vi "Benchmark SV Send  LV2012 - NI Verified - 1000 Byte - 1Var.vi"() -> ()   [LabVIEW 2019]
uses:
  <vilib>/Platform/TimedLoop/XDataNode/timing_clust.ctl
  <vilib>/Platform/TimedLoop/XDataNode/nitl_modes.ctl
  <vilib>/Platform/TimedLoop/XDataNode/wakeup.ctl
  <vilib>/platform/TimedLoop/XDataNode/XDataNode.xnode
  <vilib>/Platform/TimedLoop/XDataNode/XDNodeRunTimeDep.lvlib
panel:
  in  "Client Closed":string="The client VI closed the connection."
  in  "Stop":bool
  out "Time":u32
  out "Tries":u32
  out "Average Delay (ms)":dbl
  out "Delay (ms)":u32
  # "Overview:  Coding that exemplifies how to benchmark the communication of Shared Variables.\nRequirements: LabVIEW 2012 or compatible\nInstructions:\n1.  Run the \"Benchmark SV Receive LV2012 - NI Verified.vi\"\n2. Run this VI\n3. Watch the amount of time it takes to communicate\n4. Stop both VIs"
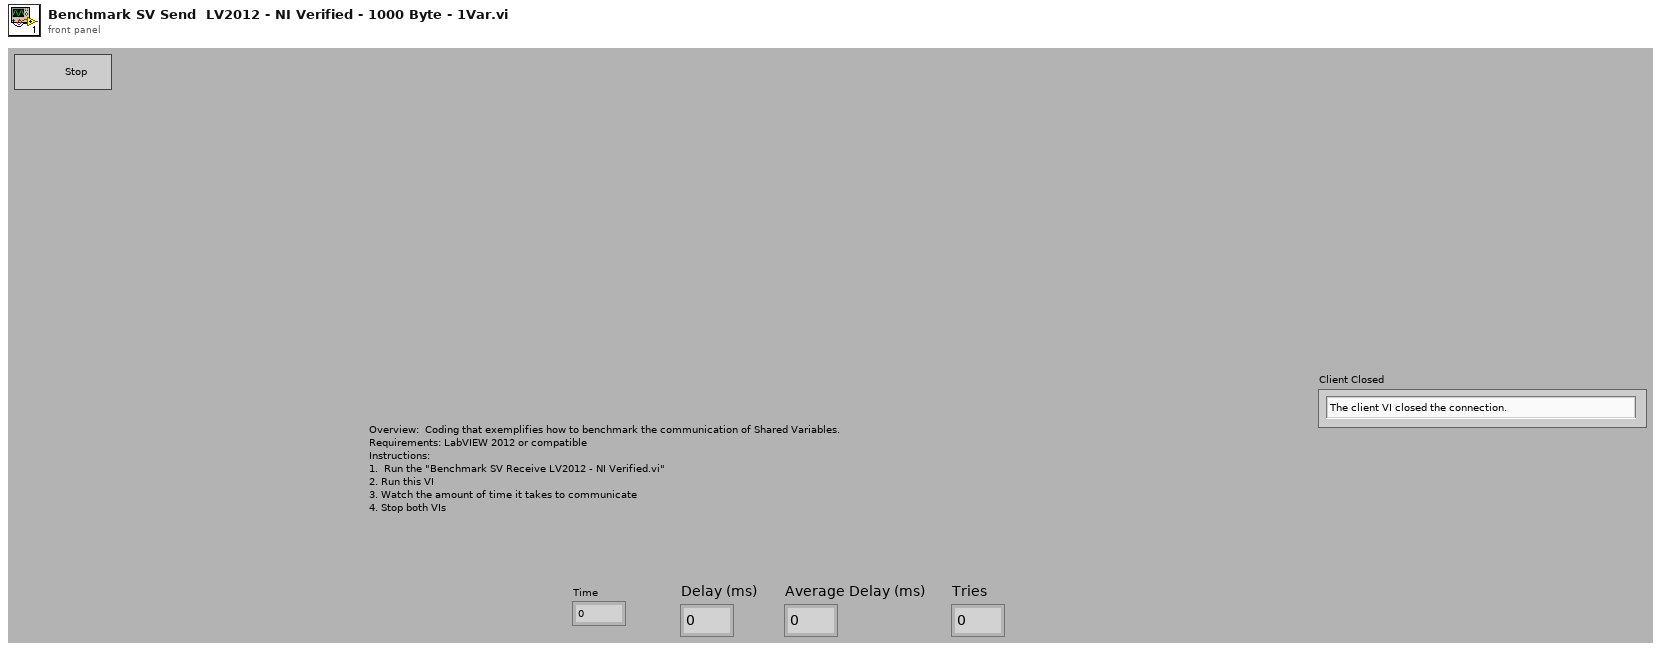
[diagram p1: front panel]
types:
  T1 = typedef "XDNodeRunTimeDep.lvlib/timing_clust.ctl" = cluster{"Expected End [f-1]":u64, "Actual End [f-1]":u64, "Finished Late? [f-1]":bool, "Expected End [i-1]":u64, "Actual End [i-1]":u64, "Finished Late? [i-1]":bool, "Expected Start [i]":u64, "Actual Start [i]":u64, "Expected Start [f]":u64, "Actual Start [f]":u64, "Source Name":string, "Structure Name":string, "Period":i64, "Deadline":i64, "Offset":i64, "Start":i64, "Priority":i32, "Timeout":i32, "Mode":T2, "Wakeup Reason":T3, "Error":errorcluster, "Source Type":string, "Secondary Source Type":string, "Global End Time":u64, "Global Start Time":u64, "Frame Duration":u64, "Iteration Duration":u64, "Assigned CPU":i32, "I/O Scan Engine Mode":u32}
  T2 = typedef "XDNodeRunTimeDep.lvlib/nitl_modes.ctl" = enum32{"No Change", "Process missed periods, maintain original phase", "Discard missed periods, maintain original phase", "Process missed periods, ignore original phase", "Discard missed periods, ignore original phase"}
  T3 = typedef "XDNodeRunTimeDep.lvlib/wakeup.ctl" = enum32{"Normal", "Aborted", "Asynchronous wakeup", "Timing source error", "Timed loop error", "Timeout"}
  T4 = cluster{i32, i32, i32, i32, i32, i32, i32, i32, i32, i32, i32, i32, i32, i32, i32, i32, i32, i32, i32, i32}
  T5 = cluster{cluster{i32, i32, i32, i32, i32, i32, i32, i32, i32, i32, i32, i32, i32, i32, i32, i32, i32, i32, i32, i32}, cluster{i32, i32, i32, i32, i32, i32, i32, i32, i32, i32, i32, i32, i32, i32, i32, i32, i32, i32, i32, i32}, cluster{i32, i32, i32, i32, i32, i32, i32, i32, i32, i32, i32, i32, i32, i32, i32, i32, i32, i32, i32, i32}, cluster{i32, i32, i32, i32, i32, i32, i32, i32, i32, i32, i32, i32, i32, i32, i32, i32, i32, i32, i32, i32}, cluster{i32, i32, i32, i32, i32, i32, i32, i32, i32, i32, i32, i32, i32, i32, i32, i32, i32, i32, i32, i32}, cluster{i32, i32, i32, i32, i32, i32, i32, i32, i32, i32, i32, i32, i32, i32, i32, i32, i32, i32, i32, i32}, cluster{i32, i32, i32, i32, i32, i32, i32, i32, i32, i32, i32, i32, i32, i32, i32, i32, i32, i32, i32, i32}, cluster{i32, i32, i32, i32, i32, i32, i32, i32, i32, i32, i32, i32, i32, i32, i32, i32, i32, i32, i32, i32}, cluster{i32, i32, i32, i32, i32, i32, i32, i32, i32, i32, i32, i32, i32, i32, i32, i32, i32, i32, i32, i32}, cluster{i32, i32, i32, i32, i32, i32, i32, i32, i32, i32, i32, i32, i32, i32, i32, i32, i32, i32, i32, i32}, cluster{i32, i32, i32, i32, i32, i32, i32, i32, i32, i32, i32, i32, i32, i32, i32, i32, i32, i32, i32, i32}, cluster{i32, i32, i32, i32, i32, i32, i32, i32, i32, i32, i32, i32, i32, i32, i32, i32, i32, i32, i32, i32}, cluster{i32, i32, i32, i32, i32, i32, i32, i32, i32, i32, i32, i32, i32, i32, i32, i32, i32, i32, i32, i32}, cluster{i32, i32, i32, i32, i32, i32, i32, i32, i32, i32, i32, i32, i32, i32, i32, i32, i32, i32, i32, i32}, cluster{i32, i32, i32, i32, i32, i32, i32, i32, i32, i32, i32, i32, i32, i32, i32, i32, i32, i32, i32, i32}, cluster{i32, i32, i32, i32, i32, i32, i32, i32, i32, i32, i32, i32, i32, i32, i32, i32, i32, i32, i32, i32}, cluster{i32, i32, i32, i32, i32, i32, i32, i32, i32, i32, i32, i32, i32, i32, i32, i32, i32, i32, i32, i32}, cluster{i32, i32, i32, i32, i32, i32, i32, i32, i32, i32, i32, i32, i32, i32, i32, i32, i32, i32, i32, i32}, cluster{i32, i32, i32, i32, i32, i32, i32, i32, i32, i32, i32, i32, i32, i32, i32, i32, i32, i32, i32, i32}, cluster{i32, i32, i32, i32, i32, i32, i32, i32, i32, i32, i32, i32, i32, i32, i32, i32, i32, i32, i32, i32}, cluster{i32, i32, i32, i32, i32, i32, i32, i32, i32, i32, i32, i32, i32, i32, i32, i32, i32, i32, i32, i32}, cluster{i32, i32, i32, i32, i32, i32, i32, i32, i32, i32, i32, i32, i32, i32, i32, i32, i32, i32, i32, i32}, cluster{i32, i32, i32, i32, i32, i32, i32, i32, i32, i32, i32, i32, i32, i32, i32, i32, i32, i32, i32, i32}, cluster{i32, i32, i32, i32, i32, i32, i32, i32, i32, i32, i32, i32, i32, i32, i32, i32, i32, i32, i32, i32}, cluster{i32, i32, i32, i32, i32, i32, i32, i32, i32, i32, i32, i32, i32, i32, i32, i32, i32, i32, i32, i32}, cluster{i32, i32, i32, i32, i32, i32, i32, i32, i32, i32, i32, i32, i32, i32, i32, i32, i32, i32, i32, i32}, cluster{i32, i32, i32, i32, i32, i32, i32, i32, i32, i32, i32, i32, i32, i32, i32, i32, i32, i32, i32, i32}, cluster{i32, i32, i32, i32, i32, i32, i32, i32, i32, i32, i32, i32, i32, i32, i32, i32, i32, i32, i32, i32}, cluster{i32, i32, i32, i32, i32, i32, i32, i32, i32, i32, i32, i32, i32, i32, i32, i32, i32, i32, i32, i32}, cluster{i32, i32, i32, i32, i32, i32, i32, i32, i32, i32, i32, i32, i32, i32, i32, i32, i32, i32, i32, i32}, cluster{i32, i32, i32, i32, i32, i32, i32, i32, i32, i32, i32, i32, i32, i32, i32, i32, i32, i32, i32, i32}, cluster{i32, i32, i32, i32, i32, i32, i32, i32, i32, i32, i32, i32, i32, i32, i32, i32, i32, i32, i32, i32}, cluster{i32, i32, i32, i32, i32, i32, i32, i32, i32, i32, i32, i32, i32, i32, i32, i32, i32, i32, i32, i32}, cluster{i32, i32, i32, i32, i32, i32, i32, i32, i32, i32, i32, i32, i32, i32, i32, i32, i32, i32, i32, i32}, cluster{i32, i32, i32, i32, i32, i32, i32, i32, i32, i32, i32, i32, i32, i32, i32, i32, i32, i32, i32, i32}, cluster{i32, i32, i32, i32, i32, i32, i32, i32, i32, i32, i32, i32, i32, i32, i32, i32, i32, i32, i32, i32}, cluster{i32, i32, i32, i32, i32, i32, i32, i32, i32, i32, i32, i32, i32, i32, i32, i32, i32, i32, i32, i32}, cluster{i32, i32, i32, i32, i32, i32, i32, i32, i32, i32, i32, i32, i32, i32, i32, i32, i32, i32, i32, i32}, cluster{i32, i32, i32, i32, i32, i32, i32, i32, i32, i32, i32, i32, i32, i32, i32, i32, i32, i32, i32, i32}, cluster{i32, i32, i32, i32, i32, i32, i32, i32, i32, i32, i32, i32, i32, i32, i32, i32, i32, i32, i32, i32}, cluster{i32, i32, i32, i32, i32, i32, i32, i32, i32, i32, i32, i32, i32, i32, i32, i32, i32, i32, i32, i32}, cluster{i32, i32, i32, i32, i32, i32, i32, i32, i32, i32, i32, i32, i32, i32, i32, i32, i32, i32, i32, i32}, cluster{i32, i32, i32, i32, i32, i32, i32, i32, i32, i32, i32, i32, i32, i32, i32, i32, i32, i32, i32, i32}, cluster{i32, i32, i32, i32, i32, i32, i32, i32, i32, i32, i32, i32, i32, i32, i32, i32, i32, i32, i32, i32}, cluster{i32, i32, i32, i32, i32, i32, i32, i32, i32, i32, i32, i32, i32, i32, i32, i32, i32, i32, i32, i32}, cluster{i32, i32, i32, i32, i32, i32, i32, i32, i32, i32, i32, i32, i32, i32, i32, i32, i32, i32, i32, i32}, cluster{i32, i32, i32, i32, i32, i32, i32, i32, i32, i32, i32, i32, i32, i32, i32, i32, i32, i32, i32, i32}, cluster{i32, i32, i32, i32, i32, i32, i32, i32, i32, i32, i32, i32, i32, i32, i32, i32, i32, i32, i32, i32}, cluster{i32, i32, i32, i32, i32, i32, i32, i32, i32, i32, i32, i32, i32, i32, i32, i32, i32, i32, i32, i32}, cluster{i32, i32, i32, i32, i32, i32, i32, i32, i32, i32, i32, i32, i32, i32, i32, i32, i32, i32, i32, i32}}
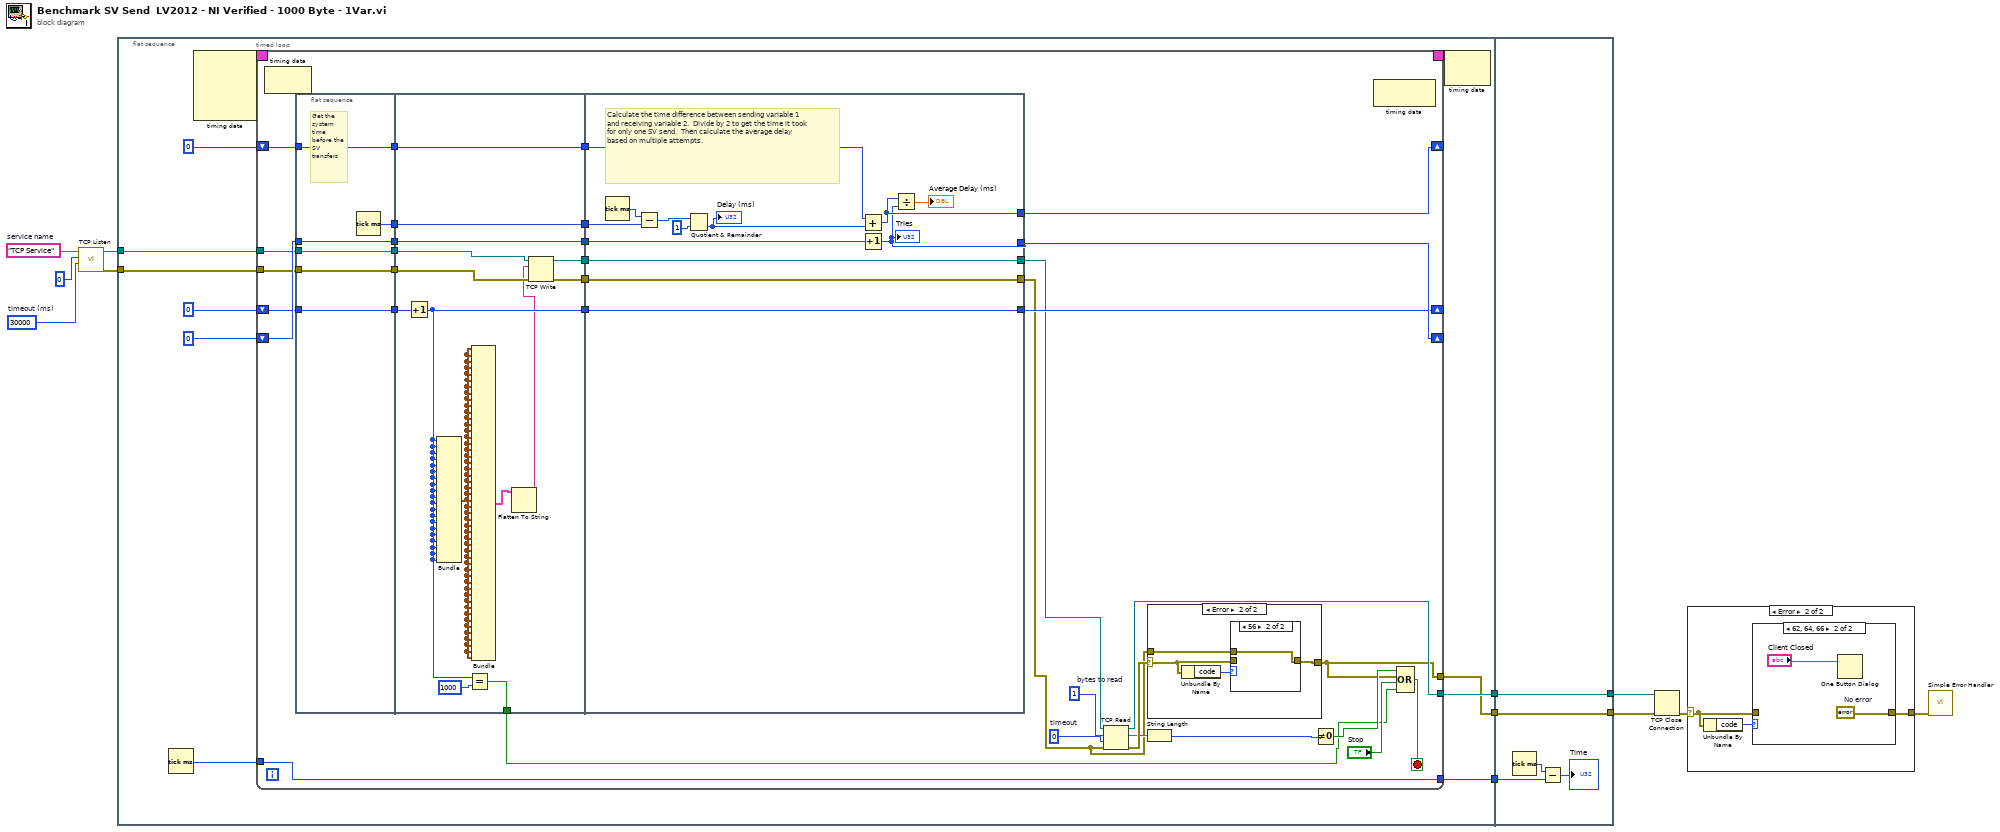
[diagram p0: block diagram]
diagram:
  w10 = "TCP Service"  # service name
  w9 = 30000  # timeout (ms)
  n1 = call <vilib>:"TCP Listen.vi"("timeout ms (wait forever: -1)"=w9, "port"=u16 0, "service name"=w10) -> ("error out"=w7:errorcluster, "connection ID"=w8:refnum<k5>)  [unwired: 4 in, 3 out]
  n2 = flat-sequence {
    tunnel: [w20] -> w12
    tunnel: w8 -> [w16]
    tunnel: w7 -> [w15]
    tunnel: [w14] -> w4
    tunnel: [w13] -> w2
    tunnel: w12 -> [w104]
    tunnel: w4 -> [w103]
    tunnel: [w103] -> w3
    tunnel: w2 -> [w102]
    tunnel: [w102] -> w1
    frame #0 {
      n3 = Tick Count (ms)() -> (millisecond timer value=w19:u32)
      n4 = node-c288() -> (w18:T1)  [unwired: 4 in]
      n5 = timed-loop {
        shift-right: [w57] -> _
        shift-left: u32 0 -> [w51]
        shift-right: [w56] -> _
        shift-left: u32 0 -> [w52]
        shift-right: [w48] -> _
        shift-left: 0 -> [w49]
        tunnel: [w43] -> w20
        tunnel: w19 -> [w43]
        timing: w18 -> [_]
        timing-out: [_] -> w17
        tunnel: w16 -> [w41]
        tunnel: w15 -> [w39]
        tunnel: [w25] -> w14
        tunnel: [w24] -> w13
        stop <- w27 stop-if-true
        w34 = 0  # timeout
        w33 = 1  # bytes to read
        n6 = node-c288() -> ()  [unwired: 1 in, 1 out]
        n7 = flat-sequence {
          tunnel: [w70] -> w55
          tunnel: [w72] -> w54
          tunnel: [w71] -> w53
          tunnel: [w69] -> w50
          tunnel: w51 -> [w72]
          tunnel: w52 -> [w71]
          tunnel: w49 -> [w69]
          tunnel: [w68] -> w42
          tunnel: w41 -> [w68]
          tunnel: [w67] -> w40
          tunnel: w39 -> [w67]
          tunnel: [w86] -> w47
          tunnel: [w85] -> w46
          tunnel: [w84] -> w45
          tunnel: w55 -> [w86]
          tunnel: w54 -> [w85]
          tunnel: w53 -> [w84]
          tunnel: w50 -> [w83]
          tunnel: [w80] -> w44
          tunnel: [w79] -> w26
          tunnel: w42 -> [w78]
          tunnel: w40 -> [w77]
          tunnel: [w76] -> w30
          tunnel: [w75] -> w28
          tunnel: w47 -> [w98]
          tunnel: [w91] -> w57
          tunnel: w46 -> [w93]
          tunnel: [w90] -> w56
          tunnel: w45 -> [w97]
          tunnel: w44 -> [w89]
          tunnel: [w89] -> w48
          tunnel: [w88] -> w31
          tunnel: w30 -> [w88]
          tunnel: [w87] -> w29
          tunnel: w28 -> [w87]
          frame #0 {
            # "Get the system time before the SV transfers"
            n8 = Tick Count (ms)() -> (millisecond timer value=w70:u32)
          }
          frame #1 {
            n9 = Increment(x=w83) -> (x+1=w80:i32)
            n10 = Bundle(w80, w80, w80, w80, w80, w80, w80, w80, w80, w80, w80, w80, w80, w80, w80, w80, w80, w80, w80, w80) -> (w81:T4)  [unwired: 1 in]
            n11 = Equal?(x=w80, y=1000) -> (x = y?=w79:bool)
            n12 = Bundle(w81, w81, w81, w81, w81, w81, w81, w81, w81, w81, w81, w81, w81, w81, w81, w81, w81, w81, w81, w81, w81, w81, w81, w81, w81, w81, w81, w81, w81, w81, w81, w81, w81, w81, w81, w81, w81, w81, w81, w81, w81, w81, w81, w81, w81, w81, w81, w81, w81, w81) -> (w74:T5)  [unwired: 1 in]
            n13 = Flatten To String(anything=w74) -> (data string=w73:string)  [unwired: 3 in, 2 out]
            n14 = TCP Write(connection ID=w78, data in=w73, error in (no error)=w77) -> (connection ID out=w76:refnum<k5>, error out=w75:errorcluster)  [unwired: 2 out]
          }
          frame #2 {
            # "Calculate the time difference between sending variable 1 and receiving variable 2.  Divide by 2 to get the time it took for only one SV send.  Then calculate the average delay based on multiple attempts."
            n15 = Tick Count (ms)() -> (millisecond timer value=w99:u32)
            n16 = Subtract(x=w99, y=w98) -> (x-y=w96:u32)
            n17 = Quotient & Remainder(x=w96, y=u32 1) -> (floor(x/y)=w94:u32)  [unwired: 1 out]
            "Delay (ms)" <- w94
            n18 = Add(x=w93, y=w94) -> (x+y=w91:u32)
            n19 = Increment(x=w97) -> (x+1=w90:u32)
            "Tries" <- w90
            n20 = Divide(x=w91, y=w90) -> (x/y=→"Average Delay (ms)":dbl)
          }
        }
        n21 = TCP Read(connection ID=w31, bytes to read=w33, error in (no error)=w29, 9:w34) -> (connection ID out=w25:refnum<k5>, data out=w36:string, error out=w38:errorcluster)  [unwired: 1 out]
        n22 = case shown="Error" w38 {
          selector: w38 -> [w58 w61]
          tunnel: [w58 w59] -> w24
          tunnel: w29 -> [_ w60]
          frame No Error {
          }
          frame Error {
            n23 = Unbundle By Name(w61) -> ("code"=w62:i32)
            n24 = case shown="56" w62 {
              tunnel: w61 -> [w63 _]
              tunnel: w60 -> [_ w64]
              tunnel: [w63 w64] -> w59
              frame Default {
              }
              frame 56 {
              }
            }
          }
        }
        n25 = String Length(string=w36) -> (length=w35:i32)
        n26 = Not Equal To 0?(x=w35) -> (x != 0?=w37:bool)
        n27 = node-c288() -> ()  [unwired: 1 in, 1 out]
        n28 = Compound Arithmetic op=OR(w37, w24, "Stop", w26) -> (w27:bool)
      }
      n29 = node-c288(w17) -> ()  [unwired: 1 out]
    }
    frame #1 {
      n30 = Tick Count (ms)() -> (millisecond timer value=w106:u32)
      n31 = Subtract(x=w106, y=w104) -> (x-y=→"Time":u32)
    }
  }
  n32 = TCP Close Connection(connection ID=w3, error in (no error)=w1) -> (error out=w6:errorcluster)  [unwired: 2 out]
  n33 = case shown="Error" w6 {
    selector: w6 -> [w107 w109]
    tunnel: [w107 w108] -> w5
    frame No Error {
    }
    frame Error {
      n34 = Unbundle By Name(w109) -> ("code"=w110:i32)
      n35 = case shown="62, 64, 66" w110 {
        tunnel: w109 -> [w111 _]
        tunnel: [w111 w113] -> w108
        frame Default {
        }
        frame 62, 64, 66 {
          w113 = errorcluster {"status"=FALSE, "code"=0, "source"=""}  # No error
          n36 = One Button Dialog(message="Client Closed") -> ()  [unwired: 1 in, 1 out]
        }
      }
    }
  }
  n37 = call <vilib>:"Simple Error Handler.vi"("error in (no error)"=w5) -> ()  [unwired: 1 in, 8 out]
